vi "RT_Main.vi"() -> ()   [LabVIEW 2020]
uses:
  <vilib>/Platform/TimedLoop/XDataNode/timing_clust.ctl
  <vilib>/Platform/TimedLoop/XDataNode/nitl_modes.ctl
  <vilib>/Platform/TimedLoop/XDataNode/wakeup.ctl
  <vilib>/FPGAPlugInAG/cRIO-9040/niLvFpga_Open_cRIO-9040.vi
  <vilib>/Utility/error.llb/Error Cluster From Error Code.vi
  <vilib>/rvi/errors/niLvFpgaAdjustHostInterfaceError.vi
  <vilib>/FPGAPlugInAG/Dynamic/niLvFpga_Close_Dynamic.vi
  <vilib>/rvi/interface/nirviOpenFPGA/nirviOpenFPGA.xnode
  FPGA Bitfiles/depapp_FPGATarget_FPGAmain_WC8wSYHNwdY.lvbitx
  FPGA_main.vi
  <vilib>/rvi/interface/nirviReadWriteControl/nirviReadWriteControl.xnode
  <vilib>/platform/TimedLoop/XDataNode/XDataNode.xnode
  <vilib>/rvi/interface/nirviMethod/nirviMethod.xnode
  <vilib>/rvi/interface/nirviCloseFPGA/nirviCloseFPGA.xnode
  <vilib>/Platform/TimedLoop/XDataNode/XDNodeRunTimeDep.lvlib
  <vilib>/dex/Stream Element Allocation Mode.ctl
  NiFpgaLv.dll
  <vilib>/rvi/errors/niLvFpgaMergeErrorWithErrorCode.vi
  <vilib>/FPGAPlugInAG/Dynamic/niLvFpga_StopFifo_Dynamic.vi
panel:
  out "size(s) 2":i32
  out "x .or. y?":bool
  out "Actual Depth of AI FIFO":u32
  out "Numeric 2":i32
  out "Numeric":i32
  out "# elements in AI buffer":u32
  out "element out":fxp<+/-,17,5>[](array[numeric])
  out "size(s)":i32
  out "Data":i32[](array[numeric])
  out "Actual Depth of Count FIFO":u32
  out "# elements when writing RT FIFO":u32
  out "size(s) of Read Counter":i32
  out "Finished Late? [i-1]":bool
  out "# elements when reading counts":u32
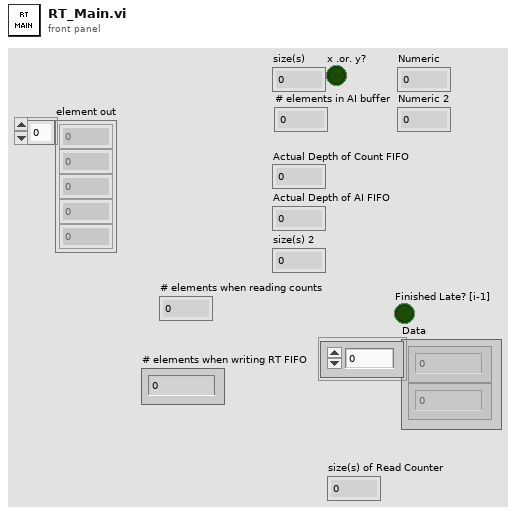
[diagram p1: front panel]
types:
  T1 = typedef "Stream Element Allocation Mode.ctl" = u32
  T2 = typedef "XDNodeRunTimeDep.lvlib/timing_clust.ctl" = cluster{"Expected End [f-1]":u64, "Actual End [f-1]":u64, "Finished Late? [f-1]":bool, "Expected End [i-1]":u64, "Actual End [i-1]":u64, "Finished Late? [i-1]":bool, "Expected Start [i]":u64, "Actual Start [i]":u64, "Expected Start [f]":u64, "Actual Start [f]":u64, "Source Name":string, "Structure Name":string, "Period":i64, "Deadline":i64, "Offset":i64, "Start":i64, "Priority":i32, "Timeout":i32, "Mode":T3, "Wakeup Reason":T4, "Error":errorcluster, "Source Type":string, "Secondary Source Type":string, "Global End Time":u64, "Global Start Time":u64, "Frame Duration":u64, "Iteration Duration":u64, "Assigned CPU":i32, "I/O Scan Engine Mode":u32}
  T3 = typedef "XDNodeRunTimeDep.lvlib/nitl_modes.ctl" = enum32{"No Change", "Process missed periods, maintain original phase", "Discard missed periods, maintain original phase", "Process missed periods, ignore original phase", "Discard missed periods, ignore original phase"}
  T4 = typedef "XDNodeRunTimeDep.lvlib/wakeup.ctl" = enum32{"Normal", "Aborted", "Asynchronous wakeup", "Timing source error", "Timed loop error", "Timeout"}
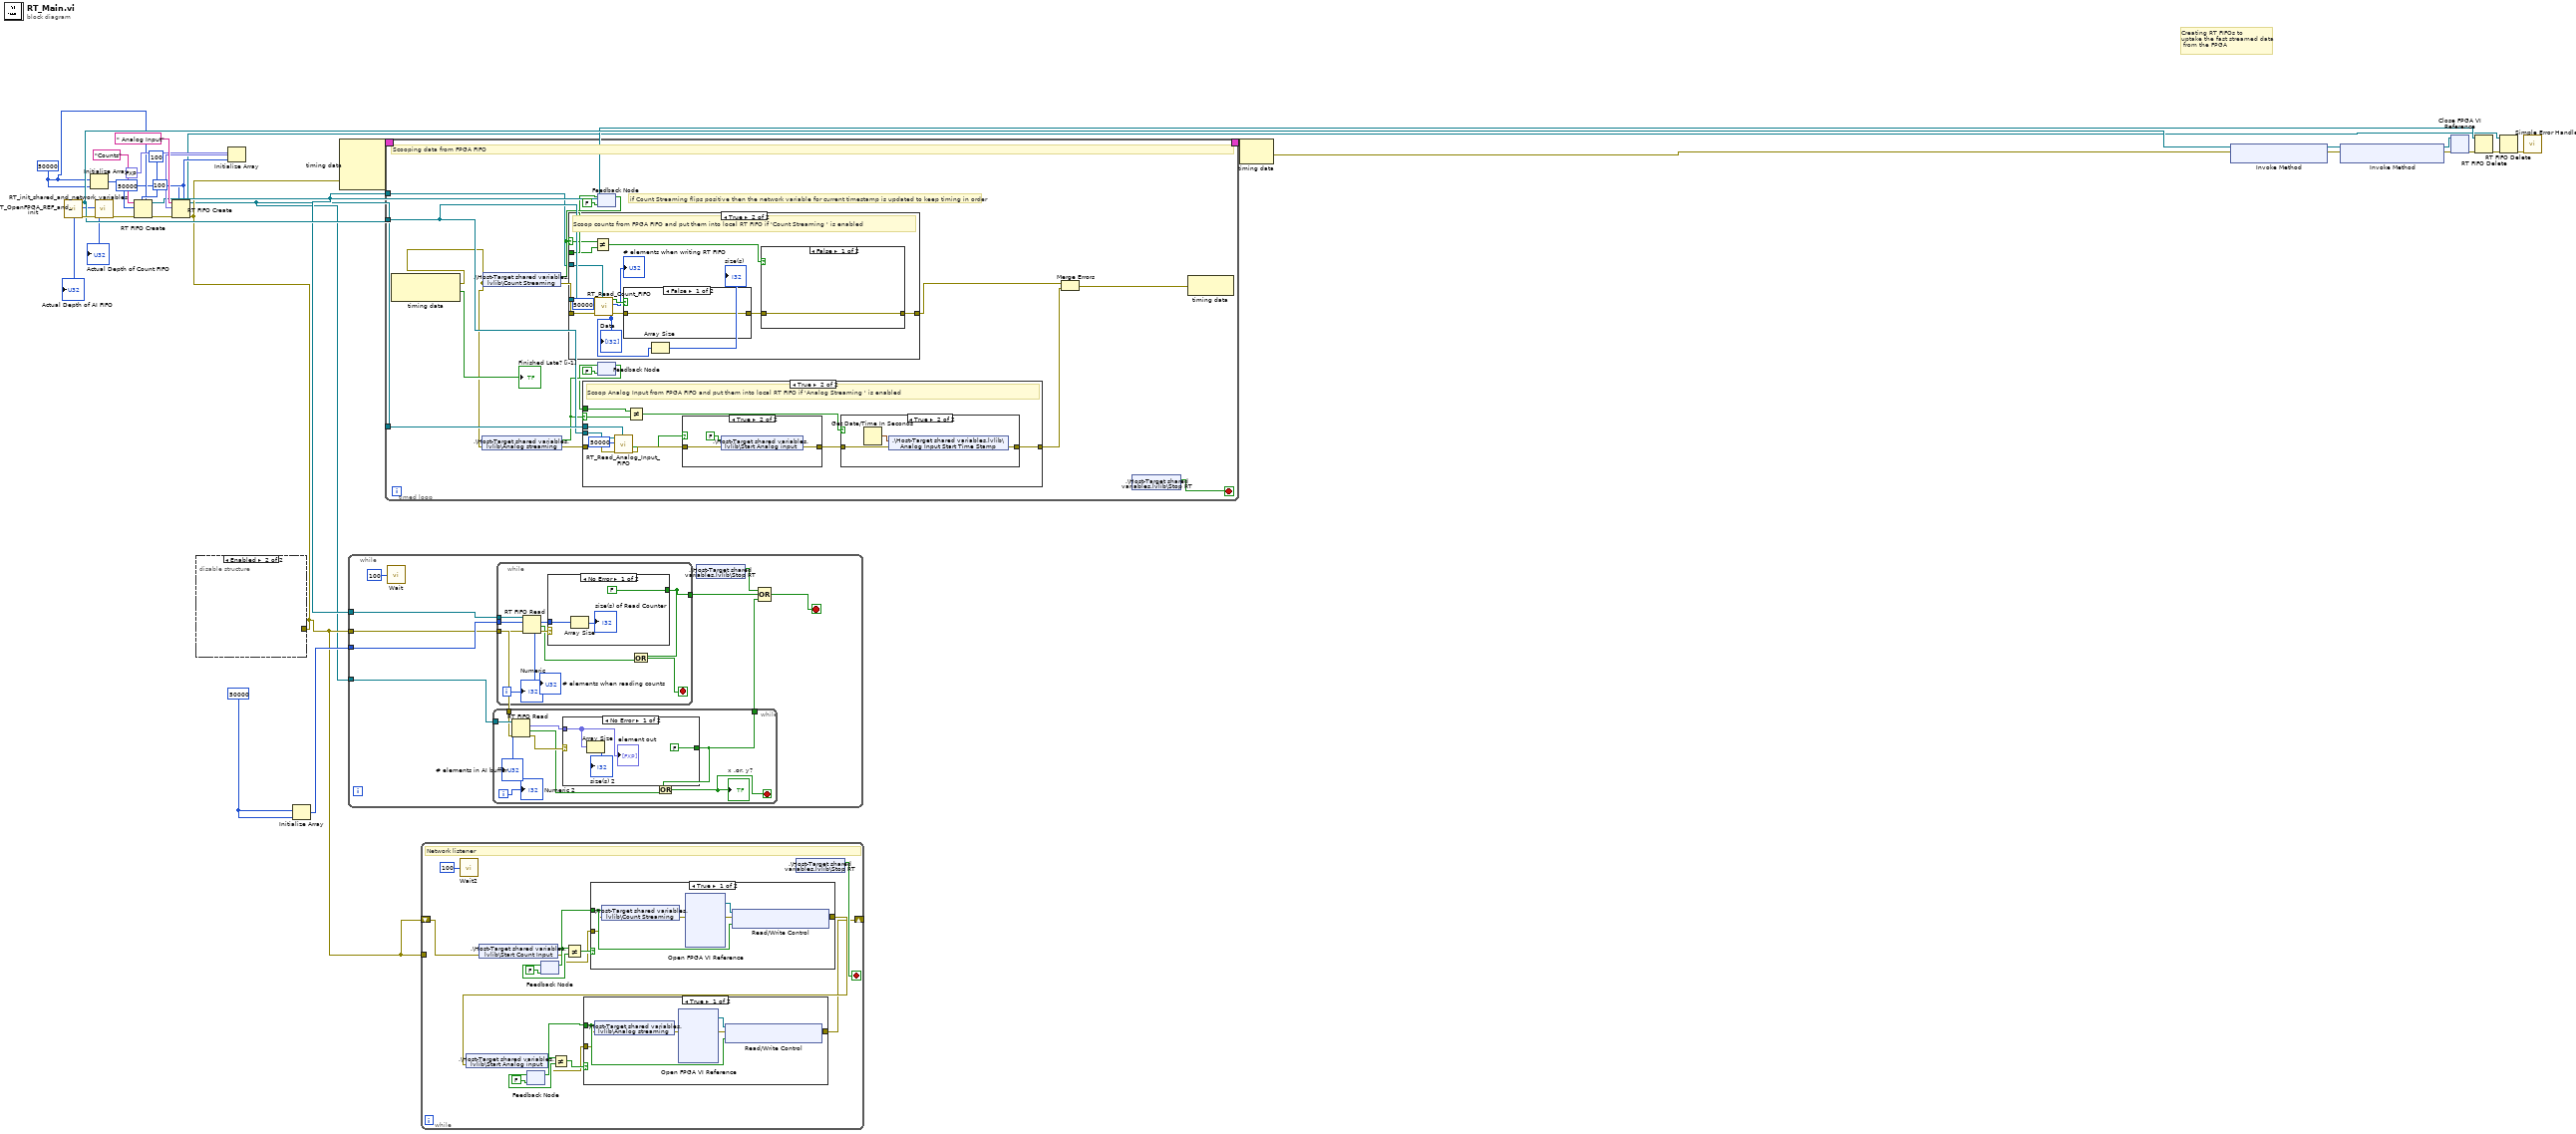
[diagram p0: block diagram]
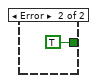
[diagram p2: hidden frame]
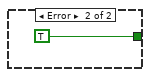
[diagram p3: hidden frame]
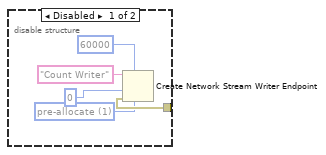
[diagram p6: hidden frame]
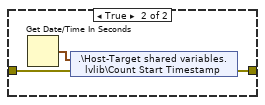
[diagram p8: hidden frame]
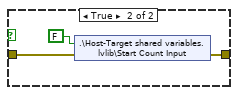
[diagram p9: hidden frame]
diagram:
  w9 = 50000
  w5 = 50000
  w4 = 50000 ("dimension size")
  # "Creating RT FIFOs to\nuptake the fast streamed data\n from the FPGA"
  n1 = call "RT_OpenFPGA_REF_and_init.vi"() -> ("error out"=w29:errorcluster, "Actual Depth of AI FIFO"=→"Actual Depth of AI FIFO":u32, "Actual Depth of Count FIFO"=→"Actual Depth of Count FIFO":u32, "Refnum out"=w18:refnum<k20>)  [unwired: 8 in]
  n2 = Initialize Array(w5, w5) -> (w6:i32[])
  n3 = call "RT_init_shared_and_network_variables.vi"("error in (no error)"=w29) -> ("error out"=w30:errorcluster)  [unwired: 10 in]
  n4 = RT FIFO Create(0:"Counts" ("name (unnamed)"), 1:w6, 3:w30, 4:u32 100 ("size (10)"), 6:w5) -> (8:w11:refnum<k33>, 11:w19:errorcluster)  [unwired: 3 in, 1 out]
  n5 = Initialize Array(fxp<+/-,17,5> 0.0, w4) -> (w23:fxp<+/-,17,5>[])
  n6 = RT FIFO Create(0:" Analog Input" ("name (unnamed)"), 1:w23, 3:w19, 4:u32 100 ("size (10)"), 6:w4) -> (8:w2:refnum<k33>, 11:w7:errorcluster)  [unwired: 3 in, 1 out]
  n7 = disable-structure shown="Enabled" {
    disable-tunnel: w7 -> [w32 _]
    frame Disabled {
      w31 = T1 1 items=["allocate as needed", "pre-allocate"] ("element allocation mode")
      n8 = Create Network Stream Writer Endpoint(6:w31, 7:60000 ("writer buffer size"), 8:w32, 9:0, 11:"Count Writer" ("writer name")) -> ()  [unwired: 2 in, 2 out]
    }
    frame Enabled {
    }
  }
  n9 = Initialize Array(w9, w9) -> (w8:i32[])
  n10 = node-c288(w7) -> (w28:T2)  [unwired: 3 in]
  n11 = while {
    tunnel: w11 -> [w40]
    tunnel: w8 -> [w39]
    tunnel: w7 -> [w37]
    tunnel: w2 -> [w38]
    stop <- w41 stop-if-true
    n12 = call "Wait"("Count(mSec)"=u32 100) -> ()  [unwired: 1 out]
    n13 = while {
      tunnel: w38 -> [w53]
      tunnel: w37 -> [w52]
      tunnel: [w51] -> w36
      i -> [w46]
      stop <- w45 stop-if-true
      n14 = RT FIFO Read(0:w53, 3:w52) -> (7:→"# elements in AI buffer":u32, 9:w49:fxp<+/-,17,5>[], 10:w47:bool, 11:w50:errorcluster)  [unwired: 2 in, 1 out]
      n15 = case shown="No Error" w50 {
        tunnel: w49 -> [w55 _]
        tunnel: [FALSE ("value") TRUE ("value")] -> w51
        frame No Error {
          n16 = Array Size(array=w55) -> (size(s)=→"size(s) 2":i32)
          "element out" <- w55
        }
        frame Error {
        }
      }
      n17 = Or(x=w51, y=w47) -> (x .or. y?=w45:bool)
      "x .or. y?" <- w45
      "Numeric 2" <- w46
    }
    n18 = while {
      tunnel: [w67] -> w43
      tunnel: w40 -> [w66]
      tunnel: w39 -> [w65]
      tunnel: w37 -> [w60]
      i -> [w58]
      stop <- w59 stop-if-true
      n19 = RT FIFO Read(0:w66, 1:w65, 3:w60) -> (7:→"# elements when reading counts":u32, 9:w63:i32[], 10:w61:bool, 11:w64:errorcluster)  [unwired: 1 in, 1 out]
      n20 = case shown="No Error" w64 {
        tunnel: [FALSE TRUE] -> w67
        tunnel: w63 -> [w69 _]
        frame No Error {
          n21 = Array Size(array=w69) -> (size(s)=→"size(s) of Read Counter":i32)
        }
        frame Error {
        }
      }
      n22 = Or(x=w67, y=w61) -> (x .or. y?=w59:bool)
      "Numeric" <- w58
    }
    n23 = shared-variable ".\\Host-Target shared variables.lvlib\\Stop RT"() -> (w42:bool)  [unwired: 1 in, 1 out]
    n24 = Compound Arithmetic op=OR(w42, w43, w36) -> (w41:bool)
  }
  n25 = timed-loop {
    timing: w28 -> [_]
    timing-out: [_] -> w27
    tunnel: w18 -> [w87]
    tunnel: w2 -> [w88]
    tunnel: w11 -> [w72]
    stop <- w76 stop-if-true
    # "if Count Streaming flips positive then the network variable for current timestamp is updated to keep timing in order"
    # "Scooping data from FPGA FIFO"
    n26 = node-c288() -> (w73:errorcluster, →"Finished Late? [i-1]":bool)  [unwired: 1 in]
    n27 = shared-variable ".\\Host-Target shared variables.lvlib\\Analog streaming"(error in=w73) -> (w79:bool, error out=w86:errorcluster)
    n28 = shared-variable ".\\Host-Target shared variables.lvlib\\Count Streaming"(error in=w73) -> (w82:bool, error out=w85:errorcluster)
    n29 = feedback-in #1(w82) -> ()
    n30 = feedback #1(FALSE ("Boolean")) -> (w80:bool)
    n31 = case shown="True" w82 {
      selector: w82 -> [_ w101]
      tunnel: w87 -> [_ w103]
      tunnel: w85 -> [w89 w102]
      tunnel: [w89 w97] -> w84
      tunnel: w80 -> [_ w100]
      tunnel: w72 -> [_ w93]
      frame False {
      }
      frame True {
        # "Scoop counts from FPGA FIFO and put them into local RT FIFO if 'Count Streaming ' is enabled"
        n32 = Not Equal?(x=w101, y=w100) -> (x != y?=w99:bool)
        n33 = call "RT_Read_Count_FIFO.vi"("rt fifo"=w93, "error in (no error)"=w102, "Elements to read"=u32 50000, "Refnum in"=w103) -> ("error out"=w95:errorcluster, "Data"=w91:i32[], "# elements 2"=→"# elements when writing RT FIFO":u32, "timed out?"=w96:bool)  [unwired: 4 in]
        "Data" <- w91
        n34 = case shown="False" w96 {
          tunnel: w95 -> [w108 w110]
          tunnel: [w108 w109] -> w98
          frame False {
          }
          frame True {
            n35 = shared-variable ".\\Host-Target shared variables.lvlib\\Start Count Input"(FALSE ("Analog streaming"), error in=w110) -> (error out=w109:errorcluster)
          }
        }
        n36 = Array Size(array=w91) -> (size(s)=→"size(s)":i32)
        n37 = case shown="False" w99 {
          tunnel: w98 -> [w104 w106]
          tunnel: [w104 w105] -> w97
          frame False {
          }
          frame True {
            n38 = Get Date/Time In Seconds() -> (seconds since 1Jan1904=w107:timestamp)
            n39 = shared-variable ".\\Host-Target shared variables.lvlib\\Count Start Timestamp"(w107, error in=w106) -> (error out=w105:errorcluster)
          }
        }
      }
    }
    n40 = feedback-in #2(w79) -> ()
    n41 = feedback #2(FALSE ("Boolean")) -> (w78:bool)
    n42 = case shown="True" w79 {
      selector: w79 -> [_ w120]
      tunnel: w87 -> [_ w123]
      tunnel: w88 -> [_ w115]
      tunnel: w86 -> [w112 w122]
      tunnel: [w112 w117] -> w83
      tunnel: w78 -> [_ w121]
      frame False {
      }
      frame True {
        # "Scoop Analog Input from FPGA FIFO and put them into local RT FIFO if 'Analog Streaming ' is enabled"
        n43 = call "RT_Read_Analog_Input_FIFO.vi"("rt fifo"=w115, "error in (no error)"=w122, "Number Of Points"=u32 50000, "Refnum in"=w123) -> ("error out"=w116:errorcluster, "timed out?"=w114:bool)  [unwired: 6 in]
        n44 = Not Equal?(x=w121, y=w120) -> (x != y?=w119:bool)
        n45 = case shown="True" w114 {
          tunnel: w116 -> [w128 w130]
          tunnel: [w128 w129] -> w118
          frame False {
          }
          frame True {
            n46 = shared-variable ".\\Host-Target shared variables.lvlib\\Start Analog input"(FALSE ("Analog streaming"), error in=w130) -> (error out=w129:errorcluster)
          }
        }
        n47 = case shown="True" w119 {
          tunnel: w118 -> [w124 w126]
          tunnel: [w124 w125] -> w117
          frame False {
          }
          frame True {
            n48 = Get Date/Time In Seconds() -> (seconds since 1Jan1904=w127:timestamp)
            n49 = shared-variable ".\\Host-Target shared variables.lvlib\\Analog Input Start Time Stamp"(w127, error in=w126) -> (error out=w125:errorcluster)
          }
        }
      }
    }
    n50 = Merge Errors(w84, w83) -> (w75:errorcluster)
    n51 = shared-variable ".\\Host-Target shared variables.lvlib\\Stop RT"() -> (w76:bool)  [unwired: 1 in, 1 out]
    n52 = node-c288(w75) -> ()  [unwired: 1 out]
  }
  n53 = while {
    tunnel: w7 -> [_]
    shift-right: [w138] -> _
    shift-left: w7 -> [w145]
    stop <- w152 stop-if-true
    # "Network listener"
    n54 = call "Wait2"("Count(mSec)"=u32 100) -> ()  [unwired: 1 out]
    n55 = shared-variable ".\\Host-Target shared variables.lvlib\\Start Count Input"(error in=w145) -> (w147:bool, error out=w146:errorcluster)
    n56 = feedback #3(FALSE ("Boolean")) -> (w144:bool)
    n57 = feedback-in #4(w147) -> ()
    n58 = feedback #4(FALSE ("Boolean")) -> (w150:bool)
    n59 = Not Equal?(x=w147, y=w150) -> (x != y?=w149:bool)
    n60 = case shown="True" w149 {
      tunnel: w147 -> [w164 _]
      tunnel: w146 -> [w161 w166]
      tunnel: [w160 w166] -> w140
      frame True {
        n61 = shared-variable ".\\Host-Target shared variables.lvlib\\Count Streaming"(w164, error in=w161) -> (error out=w165:errorcluster)
        n62 = xnode "Open FPGA VI Reference"("error in"=w165) -> ("FPGA VI Reference Out"=w163:refnum<k20>, "error out"=w162:errorcluster)  [unwired: 1 in]
        n63 = xnode "Read/Write Control"("FPGA VI Reference In"=w163, "error in"=w162, "Stream counts?"=w164) -> ("error out"=w160:errorcluster)  [unwired: 1 out]
      }
      frame False {
      }
    }
    n64 = shared-variable ".\\Host-Target shared variables.lvlib\\Start Analog input"(error in=w140) -> (w141:bool, error out=w139:errorcluster)
    n65 = feedback-in #3(w141) -> ()
    n66 = Not Equal?(x=w141, y=w144) -> (x != y?=w142:bool)
    n67 = case shown="True" w142 {
      tunnel: w141 -> [w157 _]
      tunnel: w139 -> [w154 w159]
      tunnel: [w153 w159] -> w138
      frame True {
        n68 = shared-variable ".\\Host-Target shared variables.lvlib\\Analog streaming"(w157, error in=w154) -> (error out=w158:errorcluster)
        n69 = xnode "Open FPGA VI Reference"("error in"=w158) -> ("FPGA VI Reference Out"=w156:refnum<k20>, "error out"=w155:errorcluster)  [unwired: 1 in]
        n70 = xnode "Read/Write Control"("FPGA VI Reference In"=w156, "error in"=w155, "Stream  AI"=w157) -> ("error out"=w153:errorcluster)  [unwired: 1 out]
      }
      frame False {
      }
    }
    n71 = shared-variable ".\\Host-Target shared variables.lvlib\\Stop RT"() -> (w152:bool)  [unwired: 1 in, 1 out]
  }
  n72 = node-c288(w27) -> (w17:errorcluster)
  n73 = xnode "Invoke Method"("FPGA VI Reference In"=w18, "error in"=w17) -> ("FPGA VI Reference Out"=w16:refnum<k20>, "error out"=w15:errorcluster)
  n74 = xnode "Invoke Method"("FPGA VI Reference In"=w16, "error in"=w15) -> ("FPGA VI Reference Out"=w14:refnum<k20>, "error out"=w13:errorcluster)
  n75 = xnode "Close FPGA VI Reference"("FPGA VI Reference In"=w14, "error in"=w13) -> ("error out"=w22:errorcluster)
  n76 = RT FIFO Delete(0:w11, 3:w22) -> (11:w21:errorcluster)  [unwired: 1 in]
  n77 = RT FIFO Delete(0:w2, 3:w21) -> (11:w20:errorcluster)  [unwired: 1 in]
  n78 = call <vilib>:"Simple Error Handler.vi"("error in (no error)"=w20) -> ()  [unwired: 4 in, 5 out]
